vi "Get VI Signature and GUID.vi"(8 "错误输入（无错误）":errorcluster, 11 "Path":path) -> (0 "错误输出":errorcluster, 2 "Signature:Get User Code GUID From VI File":u8[](array[numeric]), 3 "Signature:Get Signature From VI File":u8[](array[numeric]))   [LabVIEW 2012, in "Application.lvlib"]
uses:
  Application.lvlib
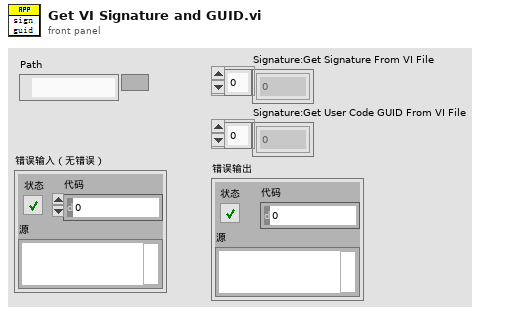
[diagram p1: front panel]
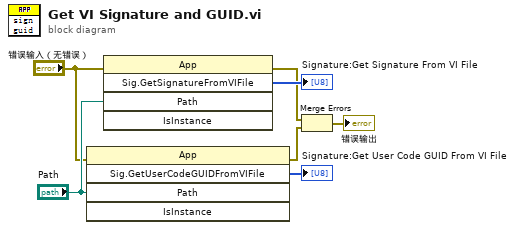
[diagram p0: block diagram]
diagram:
  n1 = invoke class="App" method="Sig.GetUserCodeGUIDFromVIFile"(error in="错误输入（无错误）", "Path"="Path") -> (error out=w3:errorcluster, "Sig.GetUserCodeGUIDFromFile"=→"Signature:Get User Code GUID From VI File":u8[])  [unwired: 3 in, 3 out]
  n2 = invoke class="App" method="Sig.GetSignatureFromVIFile"(error in="错误输入（无错误）", "Path"="Path") -> (error out=w2:errorcluster, "Sig.GetSignatureFromVIFile"=→"Signature:Get Signature From VI File":u8[])  [unwired: 3 in, 3 out]
  n3 = Merge Errors(w2, w3) -> (→"错误输出":errorcluster)
